vi "Get Base Protocol.vi"(8 "error in (no error)":errorcluster, 11 "Ethernet in":refnum<class "TCP.lvclass">) -> (0 "error out":errorcluster, 2 "Protocol out":T1, 3 "Ethernet out":refnum<class "TCP.lvclass">)   [LabVIEW 2019, in "Protocols.lvlib" / "TCP.lvclass"]
uses:
  TCP.lvclass
  Protocol Parent/Types/Base Protocol Type.ctl
  Protocol Parent/Protocol Parent.lvclass
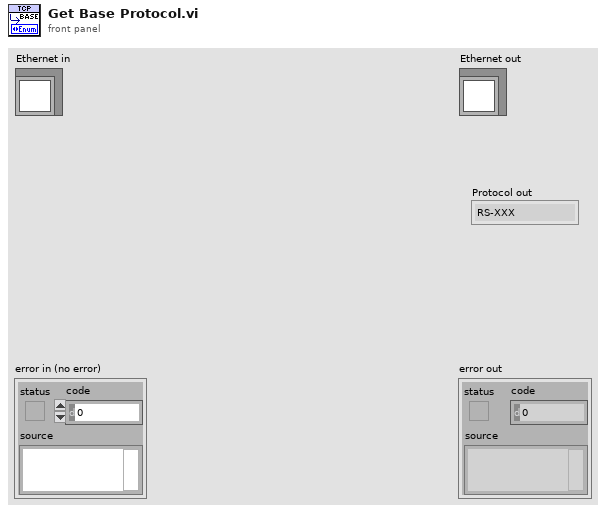
[diagram p1: front panel]
types:
  T1 = typedef "Protocols.lvlib/Protocol Parent.lvclass/Base Protocol Type.ctl" = enum16{"RS-XXX", "VISA", "TCPIP", "UDP", "GPIB ConvBox"}
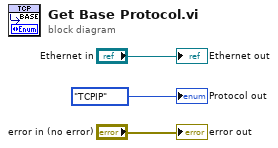
[diagram p0: block diagram]
diagram:
  "error out" <- "error in (no error)"
  "Ethernet out" <- "Ethernet in"
  "Protocol out" <- Base_Protocol_Type."TCPIP" ("Protocol out")
